vi "엣지검출.vi"(0 "Image In":T3, 1 "Color Plane (Color Plane Extraction 1)":i32(ring) items=["Red", "Green", "Blue", "Hue", "Saturation", "Luminance", "Value", "Intensity"], 2 "Filter Parameters (Filters 1)":T2={"Sigma"=1.0, "HThresh"=0.95, "LThres"=0.9000001, "WindowSize"=3}, 3 "Operation (Gray Morphology 1)":T1(ring)=enum."Dilate", 4 "Structuring Element (Gray Morphology 1)":i32[][](array[numeric])=[[1, 0, 1], [1, 0, 1], [1, 0, 1]], 7 "error in":errorcluster) -> (20 "Image Out":T3, 27 "error out":errorcluster)   [LabVIEW 2020]
uses:
  <vilib>/vision/Image Controls.llb/IMAQ Image.ctl
  <vilib>/vision/NI_Vision_Development_Module.lvlib
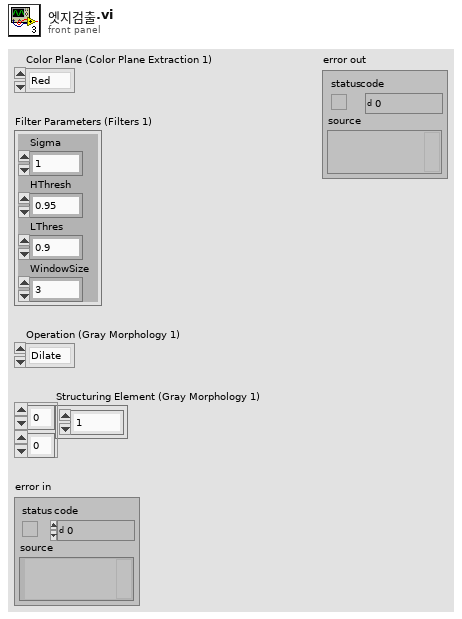
[diagram p1: front panel]
types:
  T1 = enum32{"AutoM", "Close", "Dilate", "Erode", "Gradient", "Gradient in", "Gradient out", "HitMiss", "Open", "PClose", "POpen", "Thick", "Thin"}
  T2 = cluster{"Sigma":sgl, "HThresh":sgl, "LThres":sgl, "WindowSize":i32}
  T3 = typedef "IMAQ Image.ctl" = refnum<image>
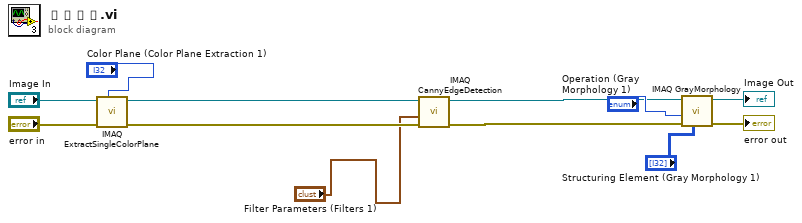
[diagram p0: block diagram]
diagram:
  n1 = call "IMAQ ExtractSingleColorPlane"("Color Plane"="Color Plane (Color Plane Extraction 1)", "error in (no error)"="error in", "Image Src"="Image In") -> ("error out"=w9:errorcluster, "Image Dst Out"=w8:T3)  [unwired: 1 in, 6 out]
  n2 = call "IMAQ CannyEdgeDetection"("Image Src"=w8, "Filter Parameters"="Filter Parameters (Filters 1)", "error in (no error)"=w9) -> ("Image Dst Out"=w3:T3, "error out"=w7:errorcluster)  [unwired: 1 in, 4 out]
  n3 = call "IMAQ GrayMorphology"("Structuring Element"="Structuring Element (Gray Morphology 1)", "error in (no error)"=w7, "Operation"="Operation (Gray Morphology 1)", "Image Src"=w3) -> ("error out"=→"error out":errorcluster, "Image Dst Out"=→"Image Out":T3)  [unwired: 3 in, 3 out]
